vi "StatePowerManagement.vi"(0 "Master State":enum16{"Normal", "Climb"}(ring)) -> ()   [LabVIEW 2020]
doc: "This VI decides whether or not power should be diverted away from non-critical subsystems in an emergency or during certain periods of the match."
uses:
  <vilib>/Rock Robotics/WPI/DriverStation/WPI_DriverStationRobotMode2.ctl
  robotoutputs.vi
  sensordata.vi
  driverdata.vi
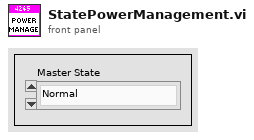
[diagram p1: front panel]
types:
  T1 = typedef "WPI_DriverStationRobotMode2.ctl" = enum16{"Autonomous Disabled", "Autonomous Enabled", "Teleop Disabled", "Teleop Enabled", "Disconnected", "Finish", "Test Disabled", "Test Enabled", "Emergency Stopped"}
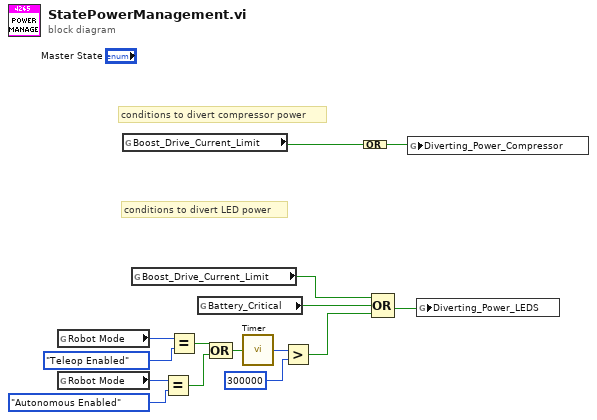
[diagram p0: block diagram]
diagram:
  # "conditions to divert LED power"
  # "conditions to divert compressor power"
  n1 = global read "driverdata.vi" "Robot Mode"() -> (w10:T1)
  n2 = global read "driverdata.vi" "Robot Mode"() -> (w7:T1)
  n3 = global read "robotoutputs.vi" "Boost_Drive_Current_Limit"() -> (w14:bool)
  n4 = global read "robotoutputs.vi" "Boost_Drive_Current_Limit"() -> (w12:bool)
  n5 = Equal?(x=w7, y=WPI_DriverStationRobotMode2."Autonomous Enabled") -> (x = y?=w5:bool)
  n6 = Equal?(x=w10, y=WPI_DriverStationRobotMode2."Teleop Enabled") -> (x = y?=w8:bool)
  n7 = global read "sensordata.vi" "Battery_Critical"() -> (w11:bool)
  n8 = Compound Arithmetic op=OR(w8, w5) -> (w2:bool)
  n9 = call "Timer.vi"("Reset Timer"=w2) -> ("Time (ms)"=w4:u32)
  n10 = Greater?(x=w4, y=u32 300000 ("x")) -> (0:w1:bool)
  n11 = Compound Arithmetic op=OR(w14) -> (w15:bool)
  n12 = Compound Arithmetic op=OR(w12, w11, w1) -> (w13:bool)
  n13 = global write "robotoutputs.vi" "Diverting_Power_Compressor"(w15) -> ()
  n14 = global write "robotoutputs.vi" "Diverting_Power_LEDS"(w13) -> ()
